vi "Concatenate table.vi"(10 "ItemNames":string[][](array[string]), 11 "ColHdrs":string[](array[string])) -> (3 "Table":string[][](array[string]))   [LabVIEW 2019]
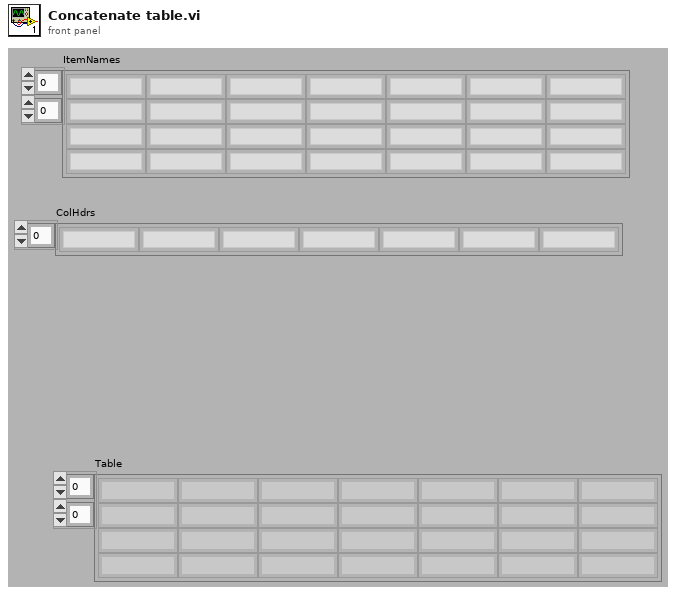
[diagram p1: front panel]
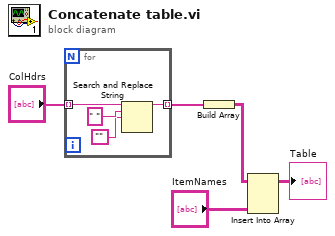
[diagram p0: block diagram]
diagram:
  n1 = for {
    tunnel: "ColHdrs" -> [w9] mode=indexing
    tunnel: [w6] -> w1 mode=indexing
    n2 = Search and Replace String(input string=w9, search string=" ", replace string="") -> (result string=w6:string)  [unwired: 1 in, 7 out]
  }
  n3 = Build Array(w1) -> (w5:string[][])
  n4 = Insert Into Array(array=w5, new element="ItemNames") -> (→"Table":string[][])  [unwired: 2 in]
